vi "Test Provoke Race Condition by Bang Writing.vi"(8 "error in (no error)":errorcluster, 11 "Test Case In":refnum<class "Configuration File Race Condition Test.lvclass">) -> (0 "error out":errorcluster, 3 "Test Case Out":refnum<class "Configuration File Race Condition Test.lvclass">)   [LabVIEW 2020, in "Configuration File Race Condition Test.lvclass"]
uses:
  Configuration File Race Condition Test.lvclass
  C:/Program Files (x86)/National Instruments/LabVIEW 2020/vi.lib/Astemes/LUnit/Test Case.lvclass
  Mock Configurable Base/Mock Configurable Base.lvclass
  <vilib>/Astemes/LUnit/Test Case.lvclass/Test Case.ctl
  01074fa8-ee8a-411d-bc8b-fc92c4f90959.vi
  <vilib>/Astemes/LUnit/Palette/Pass.vi
  <vilib>/Astemes/LUnit/Palette/Fail.vi
  <vilib>/Astemes/LUnit/Compare Variants.vi
  <vilib>/Astemes/LUnit/Describe Comparison.vi
  <vilib>/Astemes/LUnit/Set Assertion Type.vi
  <vilib>/Astemes/LUnit/Add test result.vi
  <vilib>/Astemes/LUnit/Variant to string.vi
  <vilib>/Astemes/LUnit/LUnit Record Assertion Result.vi
  <vilib>/Astemes/LUnit/LUnit Aggregate Assertion Results.vi
  <vilib>/Astemes/LUnit/Method Result/LUnit Merge Status.vi
  <vilib>/Astemes/LUnit/LUnit Concatenate result strings.vi
  <vilib>/Utility/Data Type/Get Type Information.vi
  <vilib>/Utility/LVClass/Get LV Class Name.vi
panel:
  out "text":string
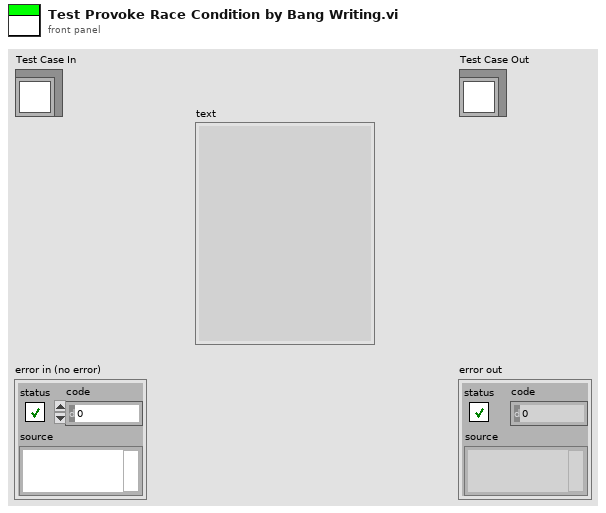
[diagram p1: front panel]
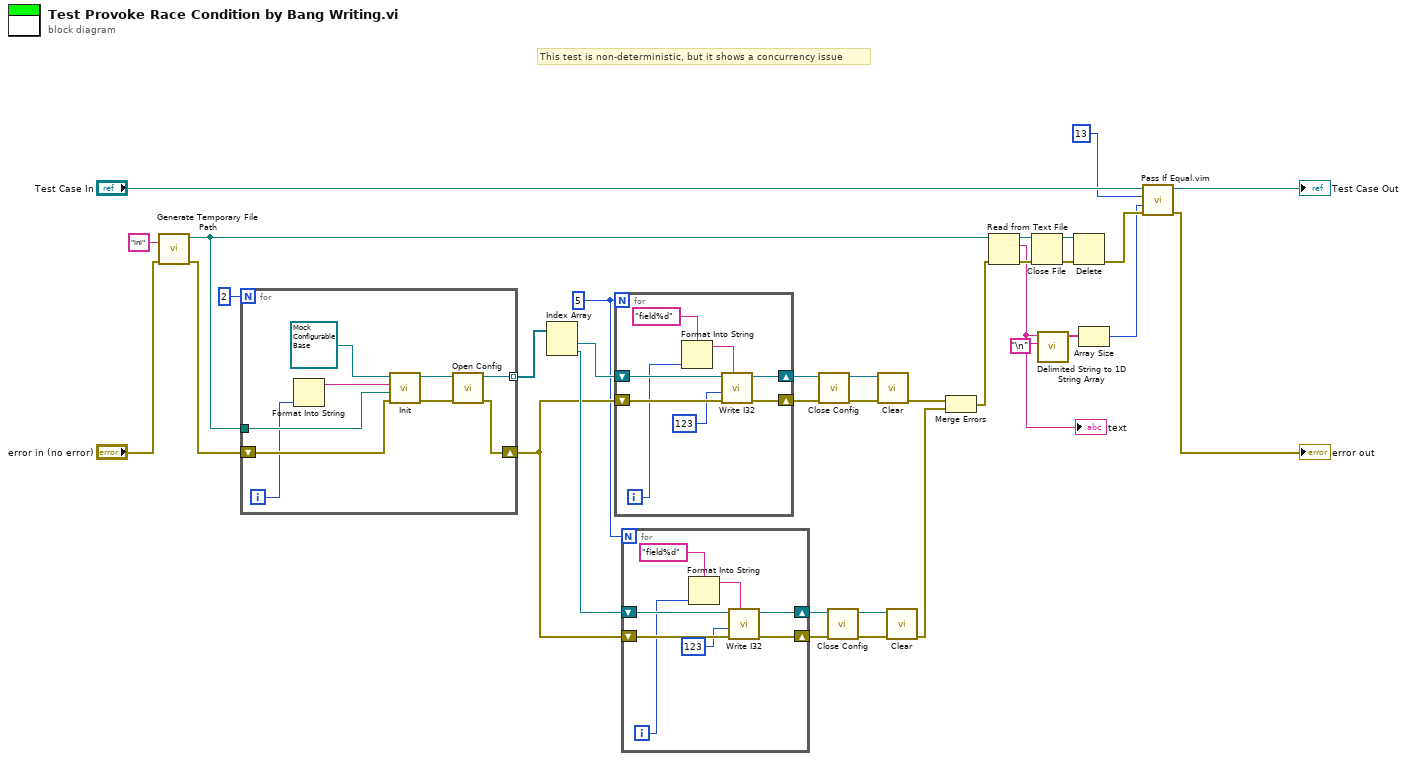
[diagram p0: block diagram]
diagram:
  w17 = 5
  # "This test is non-deterministic, but it shows a concurrency issue"
  n1 = call <vilib>:"Generate Temporary File Path.vi"("error in (no error)"="error in (no error)", "Temporary File Extension (tmp)"="ini") -> ("error out"=w30:errorcluster, "Unique Temporary File Path"=w26:path)  [unwired: 8 in]
  n2 = for {
    N: 2 -> [_]
    tunnel: w26 -> [w43]
    shift-right: [w36] -> w18
    shift-left: w30 -> [w41]
    tunnel: [w35] -> w27 mode=indexing
    i -> [w40]
    n3 = Format Into String(w40) -> (resulting string=w39:string)  [unwired: 3 in, 1 out]
    n4 = call-dynamic "Init.vi"("error in (no error)"=w41, "Config File Path"=w43, "Name"=w39, "Base In"=refnum<class "Mock Configurable Base.lvclass"> refnum ("Mock Configurable Base.lvclass")) -> ("error out"=w37:errorcluster, "Base Out"=w38:refnum<class "Mock Configurable Base.lvclass">)  [unwired: 6 in]
    n5 = call-dynamic "Open Config.vi"("error in (no error)"=w37, "Configuration File File In"=w38) -> ("error out"=w36:errorcluster, "Configuration File File Out"=w35:refnum<class "Mock Configurable Base.lvclass">)  [unwired: 8 in]
  }
  n6 = Index Array(array=w27) -> (element #1=w20:refnum<class "Mock Configurable Base.lvclass">, element #2=w19:refnum<class "Mock Configurable Base.lvclass">)  [unwired: 2 in]
  n7 = for {
    N: w17 -> [_]
    shift-right: [w44] -> w7
    shift-left: w18 -> [w51]
    shift-right: [w45] -> w9
    shift-left: w20 -> [w50]
    i -> [w46]
    n8 = Format Into String(format string="field%d" ("key"), w46) -> (resulting string=w48:string)  [unwired: 2 in, 1 out]
    n9 = call-dynamic "Write I32.vi"("key"=w48, "error in (no error)"=w51, "Value"=123, "Configuration File In"=w50) -> ("error out"=w44:errorcluster, "Configuration File Out"=w45:refnum<class "Mock Configurable Base.lvclass">)  [unwired: 6 in]
  }
  n10 = for {
    N: w17 -> [_]
    shift-right: [w52] -> w11
    shift-left: w18 -> [w59]
    shift-right: [w53] -> w14
    shift-left: w19 -> [w58]
    i -> [w54]
    n11 = Format Into String(format string="field%d" ("key"), w54) -> (resulting string=w56:string)  [unwired: 2 in, 1 out]
    n12 = call-dynamic "Write I32.vi"("key"=w56, "error in (no error)"=w59, "Value"=123, "Configuration File In"=w58) -> ("error out"=w52:errorcluster, "Configuration File Out"=w53:refnum<class "Mock Configurable Base.lvclass">)  [unwired: 6 in]
  }
  n13 = call-dynamic "Close Config.vi"("error in (no error)"=w7, "Configuration File File In"=w9) -> ("error out"=w6:errorcluster, "Configuration File File Out"=w10:refnum<class "Mock Configurable Base.lvclass">)  [unwired: 8 in]
  n14 = call-dynamic "Close Config.vi"("error in (no error)"=w11, "Configuration File File In"=w14) -> ("error out"=w12:errorcluster, "Configuration File File Out"=w15:refnum<class "Mock Configurable Base.lvclass">)  [unwired: 8 in]
  n15 = call-dynamic "Clear.vi"("error in (no error)"=w6, "Base In"=w10) -> ("error out"=w8:errorcluster)  [unwired: 9 in]
  n16 = call-dynamic "Clear.vi"("error in (no error)"=w12, "Base In"=w15) -> ("error out"=w13:errorcluster)  [unwired: 9 in]
  n17 = Merge Errors(w8, w13) -> (w16:errorcluster)
  n18 = Read from Text File(file (use dialog)=w26, error in=w16) -> (refnum out=w24:refnum<file>, text=w4:string, error out=w25:errorcluster)  [unwired: 2 in, 1 out]
  "text" <- w4
  n19 = Close File(refnum=w24, error in=w25) -> (path=w21:path, error out=w23:errorcluster)
  n20 = call <vilib>:"Delimited String to 1D String Array.vi"("delimiter"="\n", "delimited string"=w4) -> ("string array"=w3:string[])  [unwired: 9 in]
  n21 = Delete(path (use dialog)=w21, error in=w23) -> (error out=w22:errorcluster)  [unwired: 3 in, 2 out]
  n22 = Array Size(array=w3) -> (size(s)=w2:i32)
  n23 = call "Pass If Equal.vim"("error in (no error)"=w22, "Actual"=w2, "Expected"=13 ("size(s)"), "LUnit Test Case In"="Test Case In") -> ("error out"=→"error out":errorcluster, "LUnit Test Case Out"=→"Test Case Out":refnum<class "Configuration File Race Condition Test.lvclass">)  [unwired: 6 in]
